vi "Add New Message Group.vi"(8 "error in (no error)":errorcluster, 11 "Node Ptr":u64 format="%.0x") -> (0 "error out":errorcluster)   [LabVIEW 2018, in "Instrument Addon System Explorer.lvlib"]
uses:
  Instrument Addon System Explorer.lvlib
  Addon Shared/SubVIs/Constants.vi
  APIs/Scripting API/Instrument Addon Scripting API.lvlib
  Addon Shared/Instrument Addon Shared.lvlib
  <vilib>/NI Veristand/Custom Device API/Custom Device API.lvlib
panel:
  in  "Tag":string
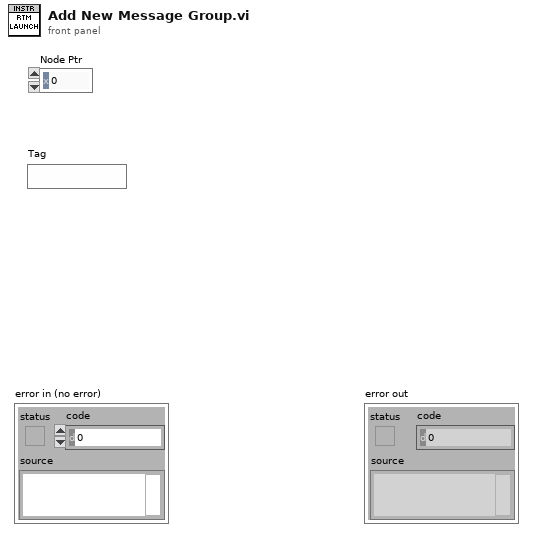
[diagram p1: front panel]
types:
  T1 = typedef "Custom Device API.lvlib/Custom Device Item Ref.ctl" = u64
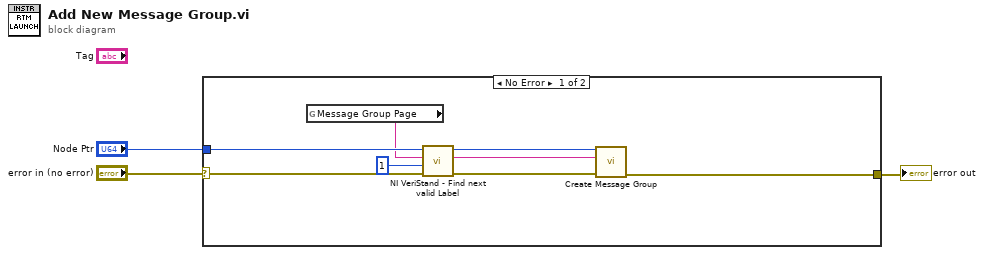
[diagram p0: block diagram]
diagram:
  n1 = case shown="No Error" "error in (no error)" {
    selector: "error in (no error)" -> [w10 w12]
    tunnel: [w11 w12] -> w2
    tunnel: "Node Ptr" -> [w8 _]
    frame No Error {
      n2 = global read "Constants.vi" "Message Group Page"() -> (w7:string)
      n3 = call <vilib>:"NI VeriStand - Find next valid Label.vi"("error in (no error)"=w10, "Start Value (1)"=1, "Label"=w7, "Item Ref in"=w8) -> ("error out"=w9:errorcluster, "Label out"=w6:string, "Item Ref out"=w5:T1)  [unwired: 3 in, 2 out]
      n4 = call "Create Message Group.vi"("error in (no error)"=w9, "message group name"=w6, "instrument addon refnum in"=w5) -> ("error out"=w11:errorcluster)  [unwired: 6 in, 2 out]
    }
    frame Error {
    }
  }
  "error out" <- w2
